vi "OAT Even Time or Speed Segment (Even Angle, N Channels).vi"(0 "even-angle signals":cluster{"r0":dbl, "dr":dbl, "Y":dbl[]}[](array[cluster]) {"r0" format="%.2p"; "dr" format="%.2p"; "Y" format="%.2f"}, 1 "segment unit":u16(ring) items=["Time (s)", "Speed (RPM)"], 2 "reset? (F)":bool, 5 "even-angle channel info":T1[](array[typedef]) {"channel info"."pregain" format="%.2f"; "channel info"."weighting filter" items=["Linear", "A-weighting", "B-weighting", "C-weighting", "ITU-R 468-4", "Dolby", "CCITT", "C-message", "Wb", "Wc", "Wd", "We", "Wf", "Wh", "Wj", "Wk", "Wm", "AES17 20 kHz lowpass", "AES17 40 kHz lowpass", "AES17 20 kHz highpass", "AES17 40 kHz highpass"]; "channel info"."dB reference" format="%^.1e"; "channel info"."engineering units" items=["custom..."=0, "V"=1, "A"=21, "C"=30, "pC"=31, "s"=32, "-"=29, "Pa"=2, "N"=20, "g"=3, "m/s^2"=4, "m/s"=5, "m"=6, "mm/s"=12, "mm"=13, "micron/s"=14, "micron"=15, "in/s^2"=7, "in/s"=8, "in"=9, "mil/s"=10, "mil"=11, "rad/s^2"=16, "rad/s"=17, "rad"=18, "deg/s^2"=26, "deg/s"=27, "deg"=28, "RPM"=22, "cycle/s^2"=23, "Hz"=24, "cycle"=25, "strain"=19]; "channel info"."sensor sensitivity" format="%#_5f"}, 7 "speed profile":T7 {"speed [RPM]" format="%.2f"; "time [s]" format="%.2f"}, 9 "pulse/revolution (1)":i32=1, 11 "error in (no error)":errorcluster, 12 "segment settings":cluster{"start":dbl, "end":dbl, "step size":dbl} {"step size" format="%.2f"; "end" min=0.0 format="%.2f"; "start" min=0.0 format="%.2f"}, 13 "segment block size":i32=128 min=2) -> (4 "even-angle signals out":cluster{"r0":dbl, "dr":dbl, "Y":dbl[]}[](array[cluster]) {"r0" format="%.2p"; "dr" format="%.2p"; "Y" format="%.2f"}, 6 "dup even-angle channel info":T1[](array[typedef]) {"channel info"."pregain" format="%.2f"; "channel info"."weighting filter" items=["Linear", "A-weighting", "B-weighting", "C-weighting", "ITU-R 468-4", "Dolby", "CCITT", "C-message", "Wb", "Wc", "Wd", "We", "Wf", "Wh", "Wj", "Wk", "Wm", "AES17 20 kHz lowpass", "AES17 40 kHz lowpass", "AES17 20 kHz highpass", "AES17 40 kHz highpass"]; "channel info"."dB reference" format="%^.1e"; "channel info"."engineering units" items=["custom..."=0, "V"=1, "A"=21, "C"=30, "pC"=31, "s"=32, "-"=29, "Pa"=2, "N"=20, "g"=3, "m/s^2"=4, "m/s"=5, "m"=6, "mm/s"=12, "mm"=13, "micron/s"=14, "micron"=15, "in/s^2"=7, "in/s"=8, "in"=9, "mil/s"=10, "mil"=11, "rad/s^2"=16, "rad/s"=17, "rad"=18, "deg/s^2"=26, "deg/s"=27, "deg"=28, "RPM"=22, "cycle/s^2"=23, "Hz"=24, "cycle"=25, "strain"=19]; "channel info"."sensor sensitivity" format="%#_5f"}, 8 "new signal available?":bool, 10 "current segment status":T6, 14 "actual segment settings":T5 {"actual step size" format="%.2f"; "actual end" min=0.0 format="%.2f"; "actual start" min=0.0 format="%.2f"}, 15 "error out":errorcluster)   [LabVIEW 2017, in "SoundVib_OAUtility.lvlib"]
doc: "Divides an input signal into even-time segments or even-speed intervals. The input signal of this VI can be an even-angle signal or an XY signal. When you use this VI to divide an XY signal, the XY signal can be only the output of the OAT Order Magnitude and Phase VI or OAT Overall Level Plot VI. Wire data to the <B>even-angle signal</B> input to determine the polymorphic instance to use or manually select the instance."
uses:
  <vilib>/addons/Sound and Vibration/Order Analysis/Utility/SoundVib_OAUtility.lvlib
  <vilib>/addons/Sound and Vibration/Order Analysis/Tach Process/SubVIs/speed profile.ctl
  <vilib>/addons/_NISVFA/_Shared subVIs/Controls/svc_Resampled Channel Info.ctl
  <vilib>/addons/_NISVFA/_Shared subVIs/Controls/svc_Channel Info.ctl
  <vilib>/addons/_NISVFA/_Shared subVIs/Controls/svc_Engineering Units Text Ring.ctl
  <vilib>/addons/_NISVFA/_Shared subVIs/Controls/svc_Weighting Filter Text Ring.ctl
  <vilib>/addons/Sound and Vibration/Order Analysis/Tach Process/SoundVib_TachProcess.lvlib
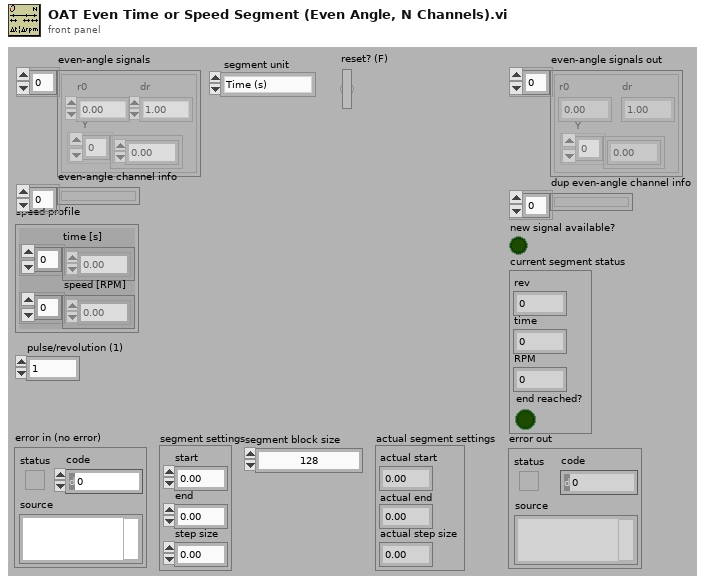
[diagram p1: front panel]
types:
  T1 = typedef "svc_Resampled Channel Info.ctl" = cluster{"channel name":string, "description":string, " channel info":T2}
  T2 = typedef "svc_Channel Info.ctl" = cluster{"sensor sensitivity":dbl, "engineering units":T3, "dB reference":dbl, "custom label":string, "weighting filter":T4, "pregain":dbl}
  T3 = typedef "svc_Engineering Units Text Ring.ctl" = u16
  T4 = typedef "svc_Weighting Filter Text Ring.ctl" = u16
  T5 = cluster{"actual start":dbl, "actual end":dbl, "actual step size":dbl}
  T6 = cluster{"rev":dbl, "time":dbl, "RPM":dbl, "end reached?":bool}
  T7 = typedef "SoundVib_TachProcess.lvlib/speed profile.ctl" = cluster{"time [s]":dbl[], "speed [RPM]":dbl[]}
  T8 = cluster{"rev":dbl, "time":dbl, "RPM":dbl, "finish?":bool}
  T9 = cluster{"last rev":dbl, "rev indice":dbl[], "time indice":dbl[], "RPM indice":dbl[]}
  T10 = cluster{"rev":dbl, "time":dbl, "RPM":dbl, "reached end?":bool}
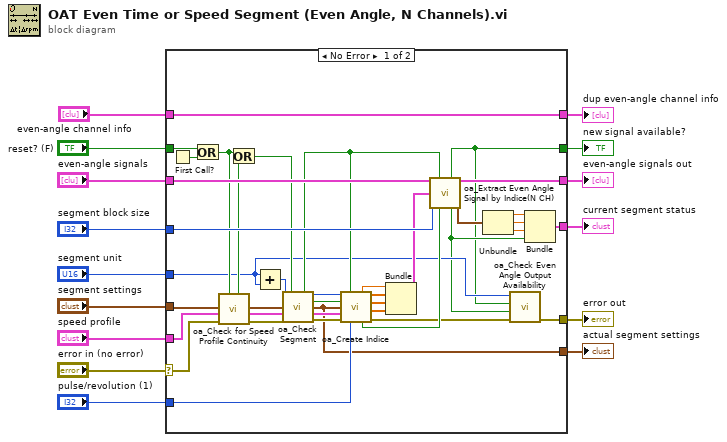
[diagram p0: block diagram]
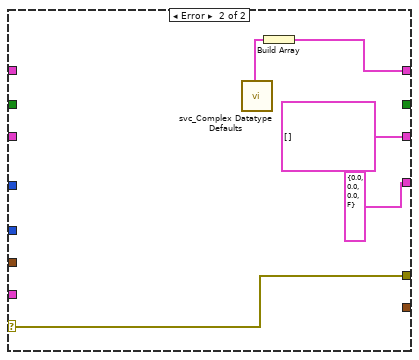
[diagram p2: hidden frame]
diagram:
  n1 = case shown="No Error" "error in (no error)" {
    selector: "error in (no error)" -> [w25 w58]
    tunnel: [w19 w58] -> w6
    tunnel: "reset? (F)" -> [w30 _]
    tunnel: "segment unit" -> [w18 _]
    tunnel: "segment settings" -> [w35 _]
    tunnel: "speed profile" -> [w34 _]
    tunnel: "even-angle channel info" -> [w53 _]
    tunnel: [w53 w54] -> w2
    tunnel: [w33 _] -> w5
    tunnel: "pulse/revolution (1)" -> [w52 _]
    tunnel: "segment block size" -> [w51 _]
    tunnel: "even-angle signals" -> [w39 _]
    tunnel: [w45 cluster{"r0":dbl, "dr":dbl, "Y":dbl[]}[] [] ("even angle signals output")] -> w3
    tunnel: [w40 T8 {"rev"=0.0, "time"=0.0, "RPM"=0.0, "finish?"=FALSE} ("current segment position")] -> w4
    tunnel: [w16 _] -> w1
    frame No Error {
      n2 = First Call?() -> (First Call?: T/F=w29:bool)
      n3 = Or(x=w30, y=w29) -> (x .or. y?=w23:bool)
      n4 = call <vilib>:"oa_Check for Speed Profile Continuity.vi"("reset in"=w23, "error in (no error)"=w25, "speed profile"=w34) -> ("error out"=w24:errorcluster, "speed profile dup"=w26:T7, "position not continuous"=w21:bool)  [unwired: 6 in]
      n5 = Or(x=w23, y=w21) -> (x .or. y?=w22:bool)
      n6 = Add(x=w18, y=w18) -> (x+y=w31:u16)
      n7 = call <vilib>:"oa_Check Segment.vi"("X axis selection"=w31, "reset?(F)"=w22, "segment position"=w35, "speed profile"=w26, "error in (no error)"=w24) -> ("reset out"=w27:bool, "X axis selection"=w32:u16, "step found?"=w36:bool, "segment position out"=w33:cluster{"start":dbl, "end":dbl, "step size":dbl}, "dul speed profile"=w37:T7, "error out"=w38:errorcluster)  [unwired: 5 in]
      n8 = call <vilib>:"oa_Create Indice.vi"("X axis selection"=w32, "reset?(F)"=w27, "step found?(F)"=w36, "steps input"=w33, "speed profile"=w37, "error in (no error)"=w38, "pulse/revolution (1)"=w52) -> ("last rev"=w50:dbl, "rev indice"=w49:dbl[], "time indice"=w48:dbl[], "RPM indice"=w47:dbl[], "reach end?"=w28:bool, "error out"=w20:errorcluster)  [unwired: 2 in, 1 out]
      n9 = Bundle("last rev"=w50, "rev indice"=w49, "time indice"=w48, "RPM indice"=w47) -> (w46:T9)  [unwired: 1 in]
      n10 = call <vilib>:"oa_Extract Even Angle Signal by Indice(N CH).vi"("even angle signals"=w39, "reset?"=w27, "trigger indices"=w46, "block size"=w51, "indices end?"=w28) -> ("new signal available?"=w16:bool, "even angle signals output"=w45:cluster{"r0":dbl, "dr":dbl, "Y":dbl[]}[], "reached end?"=w17:bool, "current position"=w44:cluster{"rev":dbl, "time":dbl, "RPM":dbl})  [unwired: 7 in]
      n11 = Unbundle(w44) -> ("rev"=w43:dbl, "time"=w42:dbl, "RPM"=w41:dbl)
      n12 = call <vilib>:"oa_Check Even Angle Output Availability.vi"("error in (no error)"=w20, "reached end?"=w17, "new signal available?"=w16, "segment unit"=w18) -> ("error out"=w19:errorcluster)  [unwired: 7 in]
      n13 = Bundle("rev"=w43, "time"=w42, "RPM"=w41, "reached end?"=w17) -> (w40:T10)  [unwired: 1 in]
    }
    frame Error {
      n14 = call <vilib>:"svc_Complex Datatype Defaults.vi"() -> ("resampled channel info"=w55:T1)  [unwired: 11 in, 8 out]
      n15 = Build Array(w55) -> (w54:T1[])
    }
  }
  "error out" <- w6
  "current segment status" <- w4
  "actual segment settings" <- w5
  "even-angle signals out" <- w3
  "dup even-angle channel info" <- w2
  "new signal available?" <- w1
